vi "Calibtarion.vi"(0 "Dwell Time (ms)":u32, 1 "V array in (V)":dbl[](array[numeric]), 2 "I array in (A)":dbl[](array[numeric]), 3 "Collected array in":dbl[][](array[numeric]), 4 "B array in (T)":dbl[](array[numeric]), 5 "Set Field (T)":dbl=0.3, 7 "dB":dbl) -> (6 "Best Linear Fit":dbl[](array[numeric]), 8 "appended array":dbl[][](array[numeric]), 9 "slope":dbl, 10 "V array out (V)":dbl[](array[numeric]), 11 "Boolean":bool, 12 "I array out (A)":dbl[](array[numeric]), 13 "intercept 2":dbl, 14 "Collected array out":dbl[][](array[numeric]), 15 "intercept":dbl, 16 "B array Out":dbl[](array[numeric]), 17 "slope 2":dbl, 18 "Best Linear Fit 2":dbl[](array[numeric]), 19 "Set Field out":dbl)   [LabVIEW 2015]
uses:
  oxford_driver/Oxford Drivers/BUSGEN.LLB/OxfordAddress.ctl
  <vilib>/Analysis/NI_AALPro.lvlib
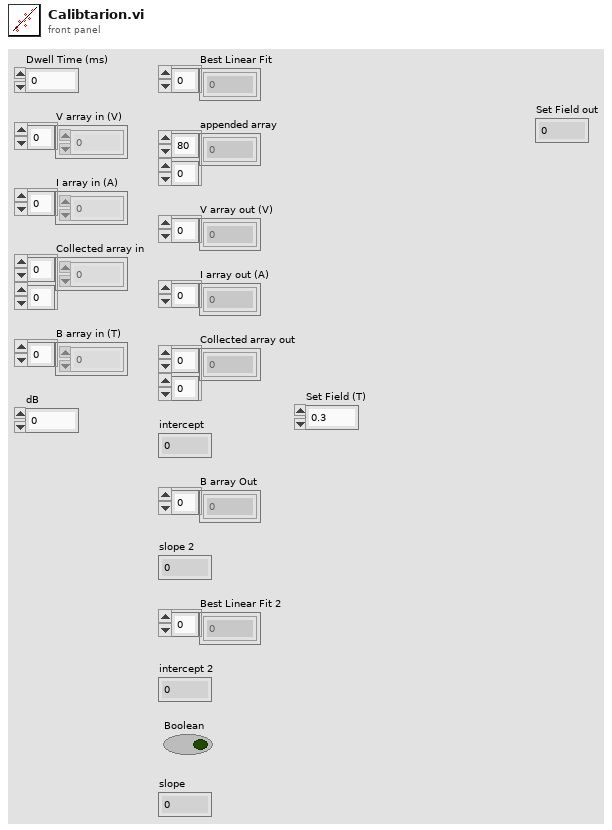
[diagram p1: front panel]
types:
  T1 = typedef "OxfordAddress.ctl" = cluster{"Com Port":i32, "ISOBUS Address":i32, "GPIB Address":i16, "Communication":enum16{"RS232", "ISOBUS", "GPIB", "Gateway"}}
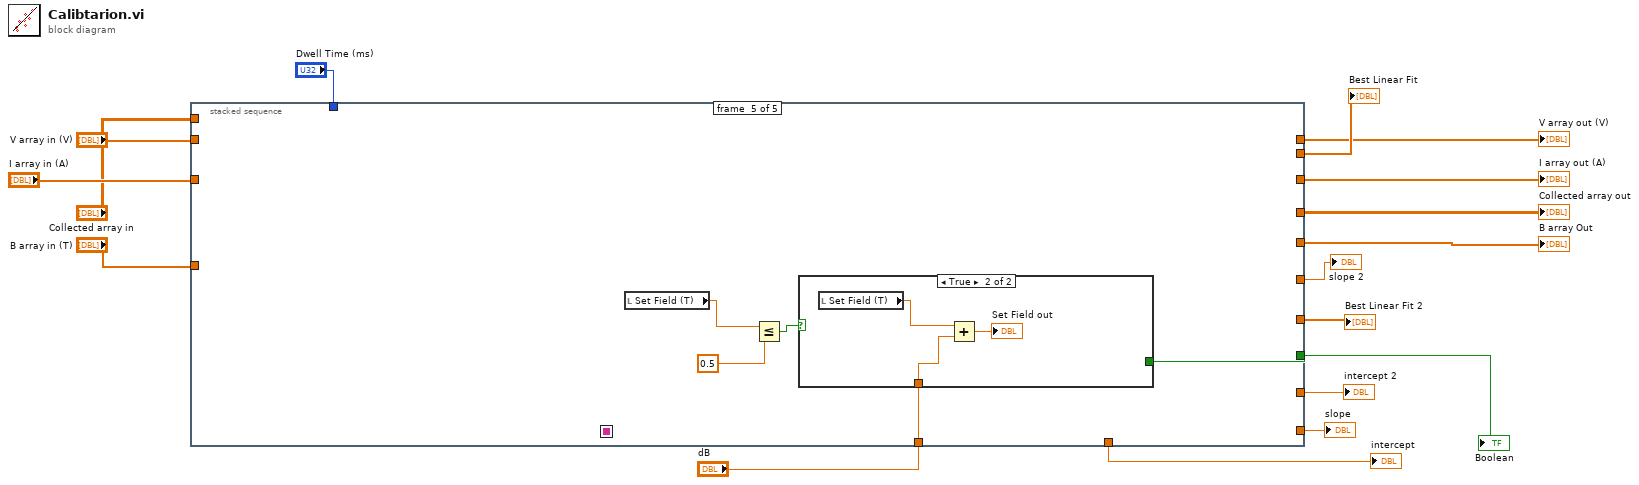
[diagram p0: block diagram]
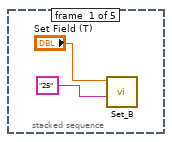
[diagram p2: hidden frame]
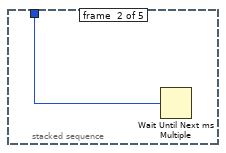
[diagram p3: hidden frame]
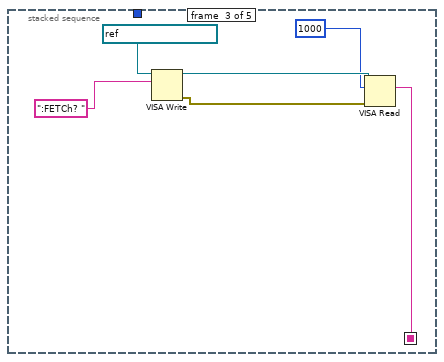
[diagram p4: hidden frame]
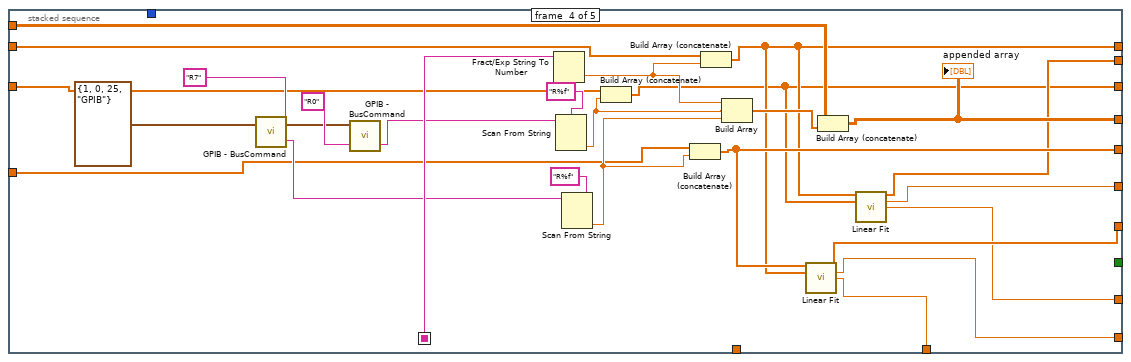
[diagram p5: hidden frame]
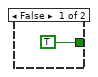
[diagram p6: hidden frame]
diagram:
  n1 = stacked-sequence {
    seq-local: [_ _ w21 _ _] -> [_ _ _ w44 _]
    tunnel: [_ _ _ w47 _] -> w3
    tunnel: "Collected array in" -> [_ _ _ w46 _]
    tunnel: [_ _ _ _ w56] -> w5
    tunnel: [_ _ _ w32 _] -> w2
    tunnel: "V array in (V)" -> [_ _ _ w41 _]
    tunnel: [_ _ _ w36 _] -> w1
    tunnel: "B array in (T)" -> [_ _ _ w39 _]
    tunnel: [_ _ _ w31 _] -> w11
    tunnel: "I array in (A)" -> [_ _ _ w37 _]
    tunnel: [_ _ _ w35 _] -> w10
    tunnel: [_ _ _ w34 _] -> w9
    tunnel: [_ _ _ w30 _] -> w12
    tunnel: [_ _ _ w29 _] -> w13
    tunnel: [_ _ _ w28 _] -> w14
    tunnel: [_ _ _ w27 _] -> w15
    tunnel: "dB" -> [_ _ _ _ w55]
    tunnel: "Dwell Time (ms)" -> [_ w20 _ _ _]
    frame #0 {
      n2 = call "Set_B.vi"("address string"="25", "Set Field (T)"="Set Field (T)") -> ()  [unwired: 9 in, 1 out]
    }
    frame #1 {
      n3 = Wait Until Next ms Multiple(millisecond multiple=w20) -> ()  [unwired: 1 out]
    }
    frame #2 {
      n4 = VISA Write(VISA resource name=refnum<visa-resource-name> "GPIB0::19::INSTR", write buffer=":FETCh? " ("data")) -> (VISA resource name out=w26:refnum<visa-resource-name>, error out=w22:errorcluster)  [unwired: 1 in, 1 out]
      n5 = VISA Read(VISA resource name=w26, byte count=u32 1000, error in (no error)=w22) -> (read buffer=w21:string)  [unwired: 3 out]
    }
    frame #3 {
      n6 = call "GPIB - BusCommand.vi"("Command"="R7" ("write buffer"), "Address"=T1 {"Com Port"=1, "ISOBUS Address"=0, "GPIB Address"=25, "Communication"=enum."GPIB"}) -> ("Reply"=w42:string, "Address(thru)"=w52:T1)
      n7 = call "GPIB - BusCommand.vi"("Command"="R0", "Address"=w52) -> ("Reply"=w43:string)  [unwired: 1 out]
      n8 = Fract/Exp String To Number(string=w44) -> (number=w33:dbl)  [unwired: 3 in, 1 out]
      n9 = Scan From String(format string="R%f" ("remaining string"), input string=w43) -> (output 1=w38:dbl)  [unwired: 3 in, 3 out]
      n10 = Scan From String(format string="R%f" ("remaining string"), input string=w42) -> (output 1=w40:dbl)  [unwired: 3 in, 3 out]
      n11 = Build Array (concatenate)(w37, w38) -> (w31:dbl[])
      n12 = Build Array (concatenate)(w39, w40) -> (w36:dbl[])
      n13 = Build Array (concatenate)(w41, w33) -> (w32:dbl[])
      n14 = Build Array(w33, w38, w40) -> (w49:dbl[])
      n15 = call <vilib>:"Linear Fit.vi"("Y"=w36, "X"=w32) -> ("Best Linear Fit"=w34:dbl[], "slope"=w28:dbl, "intercept"=w27:dbl)  [unwired: 9 in, 2 out]
      n16 = Build Array (concatenate)(w46, w49) -> (w47:dbl[][])
      "appended array" <- w47
      n17 = call <vilib>:"Linear Fit.vi"("Y"=w32, "X"=w31) -> ("Best Linear Fit"=w35:dbl[], "slope"=w30:dbl, "intercept"=w29:dbl)  [unwired: 9 in, 2 out]
    }
    frame #4 {
      n18 = local read "Set Field (T)"() -> (w54:dbl)
      n19 = Less Or Equal?(x=w54, y=0.5) -> (x <= y?=w58:bool)
      n20 = case shown="True" w58 {
        tunnel: [TRUE _] -> w56
        tunnel: w55 -> [_ w62]
        frame False {
        }
        frame True {
          n21 = local read "Set Field (T)"() -> (w61:dbl)
          n22 = Add(x=w61, y=w62) -> (x+y=→"Set Field out":dbl)
        }
      }
    }
  }
  "intercept" <- w15
  "slope" <- w14
  "intercept 2" <- w13
  "slope 2" <- w12
  "I array out (A)" <- w11
  "V array out (V)" <- w2
  "Best Linear Fit" <- w10
  "Best Linear Fit 2" <- w9
  "B array Out" <- w1
  "Boolean" <- w5
  "Collected array out" <- w3
